vi "Configure Measurement Absolute Level.vi"(0 "VISA resource name":refnum<visa-resource-name>, 1 "Ref Level Calculate Method (0: Auto Select)":i32(ring) items=["Auto Select", "Histogram", "Min/Max"], 2 "Gating (0: Screen)":u16(ring) items=["Screen", "Between Cursors", "Off"], 5 "High Ref (0 V)":dbl, 7 "Mid Ref (0 V)":dbl, 9 "Low Ref (0 V)":dbl, 11 "error in (no error)":errorcluster, 12 "Second Source Mid Ref (0 V)":dbl) -> (4 "VISA resource name out":refnum<visa-resource-name>, 15 "error out":errorcluster)   [LabVIEW 2009, in "Tektronix DPO MSO 2000 4000 Series.lvlib"]
doc: "Configures the reference levels explicitly and method an oscilloscope uses to calculate the measurement reference levels. This VI also controls the gating method for measurements."
uses:
  <instrlib>/Tektronix DPO MSO 2000 4000 Series/Tektronix DPO MSO 2000 4000 Series.lvlib
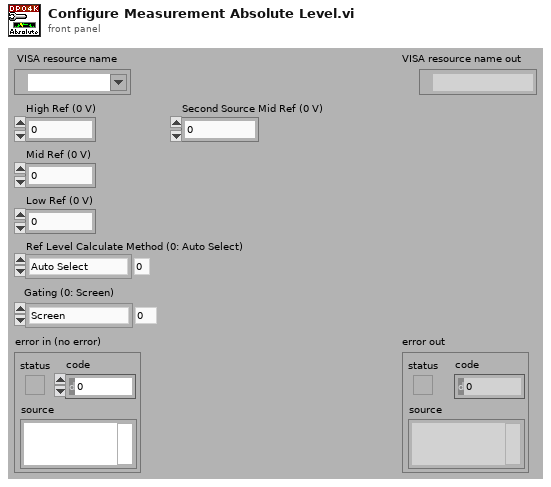
[diagram p1: front panel]
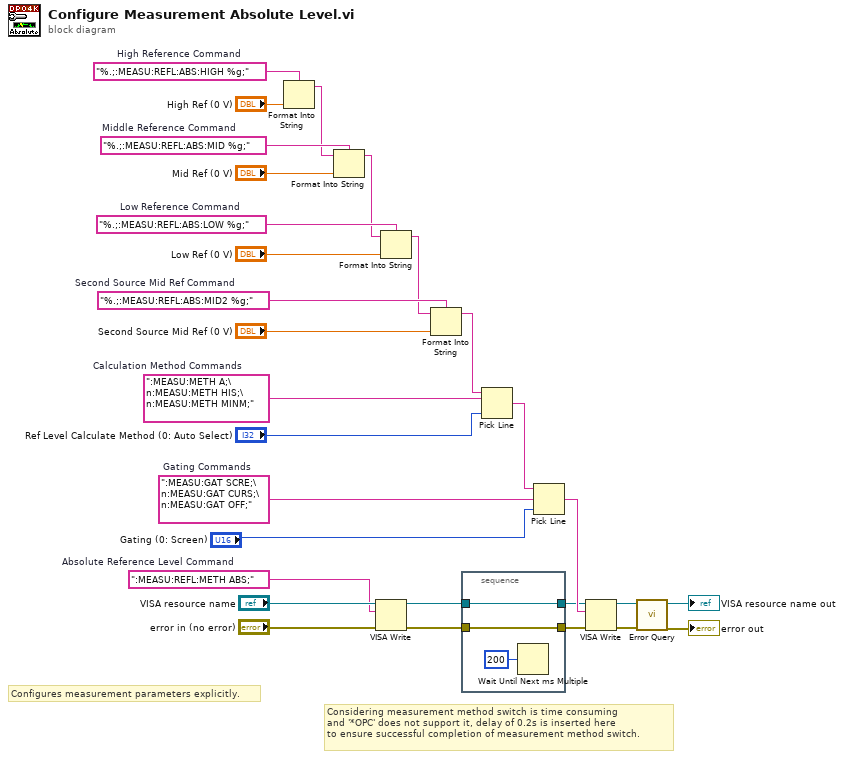
[diagram p0: block diagram]
diagram:
  w20 = ":MEASU:METH A;\n:MEASU:METH HIS;\n:MEASU:METH MINM;"  # Calculation Method Commands
  w21 = ":MEASU:GAT SCRE;\n:MEASU:GAT CURS;\n:MEASU:GAT OFF;"  # Gating Commands
  w23 = "%.;:MEASU:REFL:ABS:MID2 %g;"  # Second Source Mid Ref Command
  w25 = "%.;:MEASU:REFL:ABS:MID %g;"  # Middle Reference Command
  w27 = "%.;:MEASU:REFL:ABS:LOW %g;"  # Low Reference Command
  w29 = "%.;:MEASU:REFL:ABS:HIGH %g;"  # High Reference Command
  w6 = ":MEASU:REFL:METH ABS;"  # Absolute Reference Level Command
  # "Considering measurement method switch is time consuming\nand '*OPC' does not support it, delay of 0.2s is inserted here \nto ensure successful completion of measurement method switch."
  # "Configures measurement parameters explicitly."
  n1 = Format Into String(format string=w29, "High Ref (0 V)") -> (resulting string=w14:string)  [unwired: 2 in, 1 out]
  n2 = Format Into String(format string=w25, initial string=w14, "Mid Ref (0 V)") -> (resulting string=w13:string)  [unwired: 1 in, 1 out]
  n3 = VISA Write(VISA resource name="VISA resource name", write buffer=w6, error in (no error)="error in (no error)") -> (VISA resource name out=w5:refnum<visa-resource-name>, error out=w4:errorcluster)  [unwired: 1 out]
  n4 = Format Into String(format string=w27, initial string=w13, "Low Ref (0 V)") -> (resulting string=w12:string)  [unwired: 1 in, 1 out]
  n5 = Format Into String(format string=w23, initial string=w12, "Second Source Mid Ref (0 V)") -> (resulting string=w11:string)  [unwired: 1 in, 1 out]
  n6 = stacked-sequence {
    tunnel: w5 -> [w31]
    tunnel: [w31] -> w3
    tunnel: w4 -> [w30]
    tunnel: [w30] -> w2
    frame #0 {
      n7 = Wait Until Next ms Multiple(millisecond multiple=u32 200) -> ()  [unwired: 1 out]
    }
  }
  n8 = Pick Line(string ("")=w11, multi-line string=w20, line index="Ref Level Calculate Method (0: Auto Select)") -> (output string=w10:string)
  n9 = Pick Line(string ("")=w10, multi-line string=w21, line index="Gating (0: Screen)") -> (output string=w9:string)
  n10 = VISA Write(VISA resource name=w3, write buffer=w9, error in (no error)=w2) -> (VISA resource name out=w18:refnum<visa-resource-name>, error out=w17:errorcluster)  [unwired: 1 out]
  n11 = call <instrlib>:"Error Query.vi"("error in (no error)"=w17, "VISA resource name"=w18) -> ("error out"=→"error out":errorcluster, "VISA resource name out"=→"VISA resource name out":refnum<visa-resource-name>)  [unwired: 6 in, 2 out]
